vi "ex5 logique.vi"() -> ()   [LabVIEW 2019]
panel:
  out "IN2":bool
  out "IN1":bool
  in  "FREIN":bool
  in  "VITESSE":bool
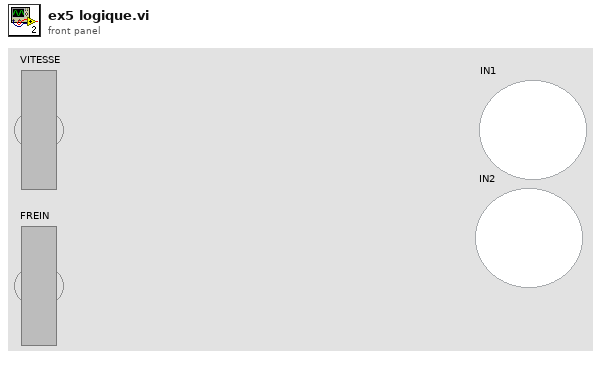
[diagram p1: front panel]
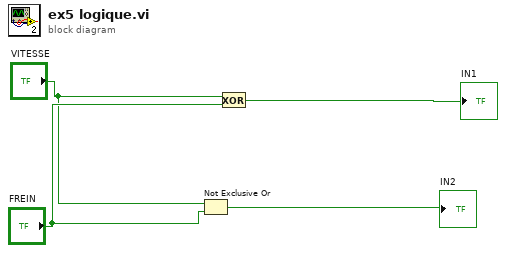
[diagram p0: block diagram]
diagram:
  n1 = Not Exclusive Or(1:"FREIN", 2:"VITESSE") -> (0:→"IN2":bool)
  n2 = Exclusive Or(1:"FREIN", 2:"VITESSE") -> (0:→"IN1":bool)
